vi "S4GUI.vi"(7 "Tab ObsEng":enum32{"Obs", "CCD modes", "Eng"}(tab)) -> ()   [LabVIEW 2018] (continued)
        n2124 = call-dynamic "Read State Machine.vi"("error in (no error)"=w4148, "Device in"=w4150) -> ("error out"=w4159:errorcluster, "State Machine.lvclass"=w4155:refnum<class "State Machine.lvclass">, "Device out"=w4156:refnum<class "Channel.lvclass">)  [unwired: 7 in]
        n2125 = call-dynamic "Read State Machine.vi"("error in (no error)"=w4165, "Device in"=w4167) -> ("error out"=w4176:errorcluster, "State Machine.lvclass"=w4172:refnum<class "State Machine.lvclass">, "Device out"=w4173:refnum<class "Channel.lvclass">)  [unwired: 7 in]
        n2126 = call-dynamic "Read State Machine.vi"("error in (no error)"=w4178, "Device in"=w4180) -> ("error out"=w4191:errorcluster, "State Machine.lvclass"=w4187:refnum<class "State Machine.lvclass">, "Device out"=w4188:refnum<class "Channel.lvclass">)  [unwired: 7 in]
        n2127 = call-dynamic "Write State.vi"("error in (no error)"=w4142, "State"=40, "State Machine in"=w4138) -> ("error out"=w4141:errorcluster, "State Machine out"=w4137:refnum<class "State Machine.lvclass">)  [unwired: 7 in]
        n2128 = call-dynamic "Write State.vi"("error in (no error)"=w4159, "State"=40, "State Machine in"=w4155) -> ("error out"=w4158:errorcluster, "State Machine out"=w4154:refnum<class "State Machine.lvclass">)  [unwired: 7 in]
        n2129 = call-dynamic "Write State.vi"("error in (no error)"=w4176, "State"=40, "State Machine in"=w4172) -> ("error out"=w4175:errorcluster, "State Machine out"=w4171:refnum<class "State Machine.lvclass">)  [unwired: 7 in]
        n2130 = call-dynamic "Write State.vi"("error in (no error)"=w4191, "State"=40, "State Machine in"=w4187) -> ("error out"=w4190:errorcluster, "State Machine out"=w4186:refnum<class "State Machine.lvclass">)  [unwired: 7 in]
        n2131 = call-dynamic "Write State Machine.vi"("error in (no error)"=w4141, "State Machine.lvclass"=w4137, "Device in"=w4139) -> ("error out"=w4135:errorcluster, "Device out"=w4136:refnum<class "Channel.lvclass">)  [unwired: 7 in]
        n2132 = call-dynamic "Write State Machine.vi"("error in (no error)"=w4158, "State Machine.lvclass"=w4154, "Device in"=w4156) -> ("error out"=w4152:errorcluster, "Device out"=w4153:refnum<class "Channel.lvclass">)  [unwired: 7 in]
        n2133 = call-dynamic "Write State Machine.vi"("error in (no error)"=w4175, "State Machine.lvclass"=w4171, "Device in"=w4173) -> ("error out"=w4169:errorcluster, "Device out"=w4170:refnum<class "Channel.lvclass">)  [unwired: 7 in]
        n2134 = call-dynamic "Write State Machine.vi"("error in (no error)"=w4190, "State Machine.lvclass"=w4186, "Device in"=w4188) -> ("error out"=w4184:errorcluster, "Device out"=w4185:refnum<class "Channel.lvclass">)  [unwired: 7 in]
        n2135 = call-dynamic "Write Channel.vi"("error in (no error)"=w4135, "Channel.lvclass"=w4136, "Acquisition in"=w4143) -> ("error out"=w4127:errorcluster, "Acquisition out"=w4128:refnum<class "Acquisition.lvclass">)  [unwired: 7 in]
        n2136 = call-dynamic "Write Channel.vi"("error in (no error)"=w4152, "Channel.lvclass"=w4153, "Acquisition in"=w4160) -> ("error out"=w4145:errorcluster, "Acquisition out"=w4144:refnum<class "Acquisition.lvclass">)  [unwired: 7 in]
        n2137 = call-dynamic "Write Channel.vi"("error in (no error)"=w4169, "Channel.lvclass"=w4170, "Acquisition in"=w4177) -> ("error out"=w4162:errorcluster, "Acquisition out"=w4161:refnum<class "Acquisition.lvclass">)  [unwired: 7 in]
        n2138 = call-dynamic "Write Channel.vi"("error in (no error)"=w4184, "Channel.lvclass"=w4185, "Acquisition in"=w4192) -> ("error out"=w4197:errorcluster, "Acquisition out"=w4198:refnum<class "Acquisition.lvclass">)  [unwired: 7 in]
        n2139 = call-dynamic "Write AcquisitionA.vi"("error in (no error)"=w4197, "Acquisition.lvclass"=w4198, "S4ACS_GUI in"=w4199) -> ("error out"=w4196:errorcluster, "S4ACS_GUI out"=w4202:refnum<class "S4GUI.lvclass">)  [unwired: 7 in]
        n2140 = call "Write AcquisitionB.vi"("error in (no error)"=w4162, "Acquisition.lvclass"=w4161, "S4ACS_GUI in"=w4202) -> ("error out"=w4195:errorcluster, "S4ACS_GUI out"=w4201:refnum<class "S4GUI.lvclass">)  [unwired: 7 in]
        n2141 = call-dynamic "Write AcquisitionC.vi"("error in (no error)"=w4145, "Acquisition.lvclass"=w4144, "S4ACS_GUI in"=w4201) -> ("error out"=w4194:errorcluster, "S4ACS_GUI out"=w4200:refnum<class "S4GUI.lvclass">)  [unwired: 7 in]
        n2142 = call-dynamic "Write AcquisitionD.vi"("error in (no error)"=w4127, "Acquisition.lvclass"=w4128, "S4ACS_GUI in"=w4200) -> ("error out"=w4193:errorcluster, "S4ACS_GUI out"=w4126:refnum<class "S4GUI.lvclass">)  [unwired: 7 in]
        n2143 = Merge Errors(w4196, w4195, w4194, w4193) -> (w4125:errorcluster)
        n2144 = call-dynamic "Write mode EXPOSE.vi"("error in (no error)"=w4125, "mode EXPOSE"=w4120, "S4GUI in"=w4126) -> ("error out"=w4123:errorcluster, "S4GUI out"=w4124:refnum<class "S4GUI.lvclass">)  [unwired: 7 in]
      }
      event "CH1on": Value Change {
        n2145 = event-data() -> ("NewVal"=w4268:bool)  [unwired: 1 in]
        n2146 = call-dynamic "Read AcquisitionA.vi"("error in (no error)"=w4282, "S4ACS_GUI in"=w4283) -> ("error out"=w4274:errorcluster, "Acquisition.lvclass"=w4279:refnum<class "Acquisition.lvclass">, "S4ACS_GUI out"=w4275:refnum<class "S4GUI.lvclass">)  [unwired: 7 in]
        n2147 = call-dynamic "Read Channel.vi"("error in (no error)"=w4274, "Acquisition in"=w4279) -> ("error out"=w4273:errorcluster, "Channel.lvclass"=w4264:refnum<class "Channel.lvclass">, "Acquisition out"=w4278:refnum<class "Acquisition.lvclass">)  [unwired: 7 in]
        n2148 = call-dynamic "Read Stream.vi"("error in (no error)"=w4273, "Server in"=w4278) -> ("error out"=w4266:errorcluster, "Stream.lvclass"=w4267:refnum<class "Stream.lvclass">, "Server out"=w4265:refnum<class "Acquisition.lvclass">)  [unwired: 7 in]
        n2149 = case shown="False" w4268 {
          selector: w4268 -> [w4284 w4306]
          tunnel: [w4290 w4310] -> w4262
          tunnel: w4267 -> [w4299 _]
          tunnel: [w4298 w4313] -> w4261
          tunnel: w4266 -> [w4285 w4307]
          tunnel: w4265 -> [w4286 w4308]
          tunnel: [w4286 w4312] -> w4260
          tunnel: w4264 -> [w4297 w4309]
          tunnel: [w4295 w4309] -> w4259
          tunnel: [w4284 w4306] -> w4263
          frame False {
            # "força FALSE nos parametros do CCD"
            n2150 = call-dynamic "Read Interface.vi"("error in (no error)"=w4285, "Channel in"=w4297) -> ("error out"=w4294:errorcluster, "Interface.lvclass"=w4288:refnum<class "Interface.lvclass">, "Channel out"=w4296:refnum<class "Channel.lvclass">)  [unwired: 7 in]
            n2151 = disable-structure shown="Enabled" {
              disable-tunnel: w4299 -> [w4303 w4305]
              disable-tunnel: [w4302 w4305] -> w4298
              disable-tunnel: [w4301 w4304] -> w4291
              disable-tunnel: w4285 -> [w4300 w4304]
              frame Disabled {
                n2152 = call-dynamic "End.vi"("error in (no error)"=w4300, "Stream in"=w4303) -> ("error out"=w4301:errorcluster, "Stream out"=w4302:refnum<class "Stream.lvclass">)  [unwired: 8 in]
              }
              frame Enabled {
              }
            }
            n2153 = call "Write Checked Params.vi"("error in (no error)"=w4294, "Checked Params"=T14 {"ACQUISITION_MODE"=FALSE, "TRIGGER_MODE"=FALSE, "READ_MODE"=FALSE, "PREAMP"=FALSE, "READOUT_RATE"=FALSE, "VERTICAL_SHIFT_SPEED"=FALSE, "EM_MODE"=FALSE, "EM_GAIN"=FALSE, "SHUTTER_MODE"=FALSE, "SHUTTER_TTL"=FALSE, "SHUTTER_OPENING_TIME"=FALSE, "SHUTTER_CLOSING_TIME"=FALSE, "VBIN"=FALSE, "HBIN"=FALSE, "INITIAL_LINE"=FALSE, "INITIAL_COLUMN"=FALSE, "FINAL_LINE"=FALSE, "FINAL_COLUMN"=FALSE, "FRAME_TRANSFER"=FALSE, "VERTICAL_CLOCK_VOLTAGE"=FALSE, "AD_CHANNEL"=FALSE}, "Interface in"=w4288) -> ("error out"=w4293:errorcluster, "Interface out"=w4287:refnum<class "Interface.lvclass">)  [unwired: 7 in]
            n2154 = call-dynamic "Write Interface.vi"("error in (no error)"=w4293, "Interface.lvclass"=w4287, "Channel in"=w4296) -> ("error out"=w4292:errorcluster, "Channel out"=w4295:refnum<class "Channel.lvclass">)  [unwired: 7 in]
            n2155 = Merge Errors(w4292, w4291) -> (w4290:errorcluster)
          }
          frame True {
            n2156 = call-dynamic "Read Stream.vi"("error in (no error)"=w4307, "Server in"=w4308) -> ("error out"=w4311:errorcluster, "Stream.lvclass"=w4314:refnum<class "Stream.lvclass">, "Server out"=w4312:refnum<class "Acquisition.lvclass">)  [unwired: 7 in]
            n2157 = disable-structure shown="Enabled" {
              disable-tunnel: w4314 -> [w4320 w4330]
              disable-tunnel: [w4319 w4330] -> w4313
              disable-tunnel: w4311 -> [w4317 w4329]
              disable-tunnel: [w4315 w4329] -> w4310
              frame Disabled {
                w4328 = FALSE ("Wait Until Done")
                n2158 = call-dynamic "Read comfile name1.vi"("error in (no error)"=w4317, "Stream in"=w4320) -> ("error out"=w4316:errorcluster, "comfile name1"=w4323:string, "Stream out"=w4318:refnum<class "Stream.lvclass">)  [unwired: 7 in]
                n2159 = call <vilib>:"Application Directory.vi"() -> ("Application Directory"=w4325:path)
                n2160 = Build Path(base path=w4325, name or relative path=w4323) -> (appended path=w4324:path)
                n2161 = Open VI Reference(vi path=w4324, error in (no error)=w4316) -> (vi reference=w4326:refnum<vi>, error out=w4327:errorcluster)  [unwired: 4 in]
                n2162 = invoke class="VI" method="Run VI"(reference=w4326, error in=w4327, "Wait until done"=w4328, "Auto Dispose Ref"=w4328) -> (reference out=w4322:refnum<vi>, error out=w4321:errorcluster)  [unwired: 1 in, 3 out]
                n2163 = call-dynamic "Write commfile ref1.vi"("error in (no error)"=w4321, "commfile ref1"=w4322, "Stream in"=w4318) -> ("error out"=w4315:errorcluster, "Stream out"=w4319:refnum<class "Stream.lvclass">)  [unwired: 7 in]
              }
              frame Enabled {
              }
            }
          }
        }
        n2164 = call-dynamic "Write Stream.vi"("error in (no error)"=w4262, "Stream.lvclass"=w4261, "Server in"=w4260) -> ("error out"=w4272:errorcluster, "Server out"=w4270:refnum<class "Acquisition.lvclass">)  [unwired: 7 in]
        n2165 = call-dynamic "Write enabled.vi"("error in (no error)"=w4272, "enabled"=w4263, "Server in"=w4270) -> ("error out"=w4271:errorcluster, "Server out"=w4269:refnum<class "Acquisition.lvclass">)  [unwired: 7 in]
        n2166 = call-dynamic "Write Channel.vi"("error in (no error)"=w4271, "Channel.lvclass"=w4259, "Acquisition in"=w4269) -> ("error out"=w4277:errorcluster, "Acquisition out"=w4276:refnum<class "Acquisition.lvclass">)  [unwired: 7 in]
        n2167 = call-dynamic "Write AcquisitionA.vi"("error in (no error)"=w4277, "Acquisition.lvclass"=w4276, "S4ACS_GUI in"=w4275) -> ("error out"=w4280:errorcluster, "S4ACS_GUI out"=w4281:refnum<class "S4GUI.lvclass">)  [unwired: 7 in]
      }
      event "CH2on": Value Change {
        n2168 = event-data() -> ("NewVal"=w4332:bool)  [unwired: 1 in]
        n2169 = call "Read AcquisitionB.vi"("error in (no error)"=w4354, "S4ACS_GUI in"=w4355) -> ("error out"=w4346:errorcluster, "Acquisition.lvclass"=w4351:refnum<class "Acquisition.lvclass">, "S4ACS_GUI out"=w4347:refnum<class "S4GUI.lvclass">)  [unwired: 7 in]
        n2170 = call-dynamic "Read Channel.vi"("error in (no error)"=w4346, "Acquisition in"=w4351) -> ("error out"=w4345:errorcluster, "Channel.lvclass"=w4340:refnum<class "Channel.lvclass">, "Acquisition out"=w4350:refnum<class "Acquisition.lvclass">)  [unwired: 7 in]
        n2171 = call-dynamic "Read Stream.vi"("error in (no error)"=w4345, "Server in"=w4350) -> ("error out"=w4336:errorcluster, "Stream.lvclass"=w4333:refnum<class "Stream.lvclass">, "Server out"=w4338:refnum<class "Acquisition.lvclass">)  [unwired: 7 in]
        n2172 = case shown="False" w4332 {
          selector: w4332 -> [w4356 w4378]
          tunnel: [w4362 w4382] -> w4335
          tunnel: w4333 -> [w4371 _]
          tunnel: [w4370 w4385] -> w4334
          tunnel: w4336 -> [w4357 w4379]
          tunnel: w4338 -> [w4358 w4380]
          tunnel: [w4358 w4384] -> w4337
          tunnel: w4340 -> [w4369 w4381]
          tunnel: [w4367 w4381] -> w4339
          tunnel: [w4356 w4378] -> w4331
          frame False {
            # "força FALSE nos parametros do CCD"
            n2173 = call-dynamic "Read Interface.vi"("error in (no error)"=w4357, "Channel in"=w4369) -> ("error out"=w4366:errorcluster, "Interface.lvclass"=w4360:refnum<class "Interface.lvclass">, "Channel out"=w4368:refnum<class "Channel.lvclass">)  [unwired: 7 in]
            n2174 = disable-structure shown="Enabled" {
              disable-tunnel: w4371 -> [w4375 w4377]
              disable-tunnel: [w4374 w4377] -> w4370
              disable-tunnel: [w4373 w4376] -> w4363
              disable-tunnel: w4357 -> [w4372 w4376]
              frame Disabled {
                n2175 = call-dynamic "End.vi"("error in (no error)"=w4372, "Stream in"=w4375) -> ("error out"=w4373:errorcluster, "Stream out"=w4374:refnum<class "Stream.lvclass">)  [unwired: 8 in]
              }
              frame Enabled {
              }
            }
            n2176 = call "Write Checked Params.vi"("error in (no error)"=w4366, "Checked Params"=T14 {"ACQUISITION_MODE"=FALSE, "TRIGGER_MODE"=FALSE, "READ_MODE"=FALSE, "PREAMP"=FALSE, "READOUT_RATE"=FALSE, "VERTICAL_SHIFT_SPEED"=FALSE, "EM_MODE"=FALSE, "EM_GAIN"=FALSE, "SHUTTER_MODE"=FALSE, "SHUTTER_TTL"=FALSE, "SHUTTER_OPENING_TIME"=FALSE, "SHUTTER_CLOSING_TIME"=FALSE, "VBIN"=FALSE, "HBIN"=FALSE, "INITIAL_LINE"=FALSE, "INITIAL_COLUMN"=FALSE, "FINAL_LINE"=FALSE, "FINAL_COLUMN"=FALSE, "FRAME_TRANSFER"=FALSE, "VERTICAL_CLOCK_VOLTAGE"=FALSE, "AD_CHANNEL"=FALSE}, "Interface in"=w4360) -> ("error out"=w4365:errorcluster, "Interface out"=w4359:refnum<class "Interface.lvclass">)  [unwired: 7 in]
            n2177 = call-dynamic "Write Interface.vi"("error in (no error)"=w4365, "Interface.lvclass"=w4359, "Channel in"=w4368) -> ("error out"=w4364:errorcluster, "Channel out"=w4367:refnum<class "Channel.lvclass">)  [unwired: 7 in]
            n2178 = Merge Errors(w4364, w4363) -> (w4362:errorcluster)
          }
          frame True {
            n2179 = call-dynamic "Read Stream.vi"("error in (no error)"=w4379, "Server in"=w4380) -> ("error out"=w4383:errorcluster, "Stream.lvclass"=w4386:refnum<class "Stream.lvclass">, "Server out"=w4384:refnum<class "Acquisition.lvclass">)  [unwired: 7 in]
            n2180 = disable-structure shown="Enabled" {
              disable-tunnel: w4386 -> [w4392 w4402]
              disable-tunnel: [w4391 w4402] -> w4385
              disable-tunnel: w4383 -> [w4389 w4401]
              disable-tunnel: [w4387 w4401] -> w4382
              frame Disabled {
                w4400 = FALSE ("Wait Until Done")
                n2181 = call-dynamic "Read comfile name1.vi"("error in (no error)"=w4389, "Stream in"=w4392) -> ("error out"=w4388:errorcluster, "comfile name1"=w4395:string, "Stream out"=w4390:refnum<class "Stream.lvclass">)  [unwired: 7 in]
                n2182 = call <vilib>:"Application Directory.vi"() -> ("Application Directory"=w4397:path)
                n2183 = Build Path(base path=w4397, name or relative path=w4395) -> (appended path=w4396:path)
                n2184 = Open VI Reference(vi path=w4396, error in (no error)=w4388) -> (vi reference=w4398:refnum<vi>, error out=w4399:errorcluster)  [unwired: 4 in]
                n2185 = invoke class="VI" method="Run VI"(reference=w4398, error in=w4399, "Wait until done"=w4400, "Auto Dispose Ref"=w4400) -> (reference out=w4394:refnum<vi>, error out=w4393:errorcluster)  [unwired: 1 in, 3 out]
                n2186 = call-dynamic "Write commfile ref1.vi"("error in (no error)"=w4393, "commfile ref1"=w4394, "Stream in"=w4390) -> ("error out"=w4387:errorcluster, "Stream out"=w4391:refnum<class "Stream.lvclass">)  [unwired: 7 in]
              }
              frame Enabled {
              }
            }
          }
        }
        n2187 = call-dynamic "Write Stream.vi"("error in (no error)"=w4335, "Stream.lvclass"=w4334, "Server in"=w4337) -> ("error out"=w4342:errorcluster, "Server out"=w4344:refnum<class "Acquisition.lvclass">)  [unwired: 7 in]
        n2188 = call-dynamic "Write enabled.vi"("error in (no error)"=w4342, "enabled"=w4331, "Server in"=w4344) -> ("error out"=w4341:errorcluster, "Server out"=w4343:refnum<class "Acquisition.lvclass">)  [unwired: 7 in]
        n2189 = call-dynamic "Write Channel.vi"("error in (no error)"=w4341, "Channel.lvclass"=w4339, "Acquisition in"=w4343) -> ("error out"=w4349:errorcluster, "Acquisition out"=w4348:refnum<class "Acquisition.lvclass">)  [unwired: 7 in]
        n2190 = call "Write AcquisitionB.vi"("error in (no error)"=w4349, "Acquisition.lvclass"=w4348, "S4ACS_GUI in"=w4347) -> ("error out"=w4352:errorcluster, "S4ACS_GUI out"=w4353:refnum<class "S4GUI.lvclass">)  [unwired: 7 in]
      }
      event "CH3 on": Value Change {
        n2191 = event-data() -> ("NewVal"=w4419:bool)  [unwired: 1 in]
        n2192 = call-dynamic "Read AcquisitionC.vi"("error in (no error)"=w4422, "S4ACS_GUI in"=w4426) -> ("error out"=w4411:errorcluster, "Acquisition.lvclass"=w4416:refnum<class "Acquisition.lvclass">, "S4ACS_GUI out"=w4412:refnum<class "S4GUI.lvclass">)  [unwired: 7 in]
        n2193 = call-dynamic "Read Channel.vi"("error in (no error)"=w4411, "Acquisition in"=w4416) -> ("error out"=w4410:errorcluster, "Channel.lvclass"=w4409:refnum<class "Channel.lvclass">, "Acquisition out"=w4415:refnum<class "Acquisition.lvclass">)  [unwired: 7 in]
        n2194 = call-dynamic "Read Stream.vi"("error in (no error)"=w4410, "Server in"=w4415) -> ("error out"=w4423:errorcluster, "Stream.lvclass"=w4427:refnum<class "Stream.lvclass">, "Server out"=w4421:refnum<class "Acquisition.lvclass">)  [unwired: 7 in]
        n2195 = case shown="False" w4419 {
          selector: w4419 -> [w4428 w4450]
          tunnel: [w4434 w4454] -> w4424
          tunnel: w4427 -> [w4443 _]
          tunnel: [w4442 w4457] -> w4425
          tunnel: w4423 -> [w4429 w4451]
          tunnel: w4421 -> [w4430 w4452]
          tunnel: [w4430 w4456] -> w4420
          tunnel: w4409 -> [w4441 w4453]
          tunnel: [w4439 w4453] -> w4408
          tunnel: [w4428 w4450] -> w4403
          frame False {
            # "força FALSE nos parametros do CCD"
            n2196 = call-dynamic "Read Interface.vi"("error in (no error)"=w4429, "Channel in"=w4441) -> ("error out"=w4438:errorcluster, "Interface.lvclass"=w4432:refnum<class "Interface.lvclass">, "Channel out"=w4440:refnum<class "Channel.lvclass">)  [unwired: 7 in]
            n2197 = disable-structure shown="Disabled" {
              disable-tunnel: w4443 -> [w4447 w4449]
              disable-tunnel: [w4446 w4449] -> w4442
              disable-tunnel: [w4445 w4448] -> w4435
              disable-tunnel: w4429 -> [w4444 w4448]
              frame Disabled {
                n2198 = call-dynamic "End.vi"("error in (no error)"=w4444, "Stream in"=w4447) -> ("error out"=w4445:errorcluster, "Stream out"=w4446:refnum<class "Stream.lvclass">)  [unwired: 8 in]
              }
              frame Enabled {
              }
            }
            n2199 = call "Write Checked Params.vi"("error in (no error)"=w4438, "Checked Params"=T14 {"ACQUISITION_MODE"=FALSE, "TRIGGER_MODE"=FALSE, "READ_MODE"=FALSE, "PREAMP"=FALSE, "READOUT_RATE"=FALSE, "VERTICAL_SHIFT_SPEED"=FALSE, "EM_MODE"=FALSE, "EM_GAIN"=FALSE, "SHUTTER_MODE"=FALSE, "SHUTTER_TTL"=FALSE, "SHUTTER_OPENING_TIME"=FALSE, "SHUTTER_CLOSING_TIME"=FALSE, "VBIN"=FALSE, "HBIN"=FALSE, "INITIAL_LINE"=FALSE, "INITIAL_COLUMN"=FALSE, "FINAL_LINE"=FALSE, "FINAL_COLUMN"=FALSE, "FRAME_TRANSFER"=FALSE, "VERTICAL_CLOCK_VOLTAGE"=FALSE, "AD_CHANNEL"=FALSE}, "Interface in"=w4432) -> ("error out"=w4437:errorcluster, "Interface out"=w4431:refnum<class "Interface.lvclass">)  [unwired: 7 in]
            n2200 = call-dynamic "Write Interface.vi"("error in (no error)"=w4437, "Interface.lvclass"=w4431, "Channel in"=w4440) -> ("error out"=w4436:errorcluster, "Channel out"=w4439:refnum<class "Channel.lvclass">)  [unwired: 7 in]
            n2201 = Merge Errors(w4436, w4435) -> (w4434:errorcluster)
          }
          frame True {
            n2202 = call-dynamic "Read Stream.vi"("error in (no error)"=w4451, "Server in"=w4452) -> ("error out"=w4455:errorcluster, "Stream.lvclass"=w4458:refnum<class "Stream.lvclass">, "Server out"=w4456:refnum<class "Acquisition.lvclass">)  [unwired: 7 in]
            n2203 = disable-structure shown="Enabled" {
              disable-tunnel: w4458 -> [w4464 w4474]
              disable-tunnel: [w4463 w4474] -> w4457
              disable-tunnel: w4455 -> [w4461 w4473]
              disable-tunnel: [w4459 w4473] -> w4454
              frame Disabled {
                w4472 = FALSE ("Wait Until Done")
                n2204 = call-dynamic "Read comfile name1.vi"("error in (no error)"=w4461, "Stream in"=w4464) -> ("error out"=w4460:errorcluster, "comfile name1"=w4467:string, "Stream out"=w4462:refnum<class "Stream.lvclass">)  [unwired: 7 in]
                n2205 = call <vilib>:"Application Directory.vi"() -> ("Application Directory"=w4469:path)
                n2206 = Build Path(base path=w4469, name or relative path=w4467) -> (appended path=w4468:path)
                n2207 = Open VI Reference(vi path=w4468, error in (no error)=w4460) -> (vi reference=w4470:refnum<vi>, error out=w4471:errorcluster)  [unwired: 4 in]
                n2208 = invoke class="VI" method="Run VI"(reference=w4470, error in=w4471, "Wait until done"=w4472, "Auto Dispose Ref"=w4472) -> (reference out=w4466:refnum<vi>, error out=w4465:errorcluster)  [unwired: 1 in, 3 out]
                n2209 = call-dynamic "Write commfile ref1.vi"("error in (no error)"=w4465, "commfile ref1"=w4466, "Stream in"=w4462) -> ("error out"=w4459:errorcluster, "Stream out"=w4463:refnum<class "Stream.lvclass">)  [unwired: 7 in]
              }
              frame Enabled {
              }
            }
          }
        }
        n2210 = call-dynamic "Write Stream.vi"("error in (no error)"=w4424, "Stream.lvclass"=w4425, "Server in"=w4420) -> ("error out"=w4406:errorcluster, "Server out"=w4407:refnum<class "Acquisition.lvclass">)  [unwired: 7 in]
        n2211 = call-dynamic "Write enabled.vi"("error in (no error)"=w4406, "enabled"=w4403, "Server in"=w4407) -> ("error out"=w4404:errorcluster, "Server out"=w4405:refnum<class "Acquisition.lvclass">)  [unwired: 7 in]
        n2212 = call-dynamic "Write Channel.vi"("error in (no error)"=w4404, "Channel.lvclass"=w4408, "Acquisition in"=w4405) -> ("error out"=w4414:errorcluster, "Acquisition out"=w4413:refnum<class "Acquisition.lvclass">)  [unwired: 7 in]
        n2213 = call-dynamic "Write AcquisitionC.vi"("error in (no error)"=w4414, "Acquisition.lvclass"=w4413, "S4ACS_GUI in"=w4412) -> ("error out"=w4417:errorcluster, "S4ACS_GUI out"=w4418:refnum<class "S4GUI.lvclass">)  [unwired: 7 in]
      }
      event "CH4 on": Value Change {
        n2214 = event-data() -> ("NewVal"=w4480:bool)  [unwired: 1 in]
        n2215 = call-dynamic "Read AcquisitionD.vi"("error in (no error)"=w4498, "S4ACS_GUI in"=w4499) -> ("error out"=w4490:errorcluster, "Acquisition.lvclass"=w4495:refnum<class "Acquisition.lvclass">, "S4ACS_GUI out"=w4491:refnum<class "S4GUI.lvclass">)  [unwired: 7 in]
        n2216 = call-dynamic "Read Channel.vi"("error in (no error)"=w4490, "Acquisition in"=w4495) -> ("error out"=w4489:errorcluster, "Channel.lvclass"=w4484:refnum<class "Channel.lvclass">, "Acquisition out"=w4494:refnum<class "Acquisition.lvclass">)  [unwired: 7 in]
        n2217 = call-dynamic "Read Stream.vi"("error in (no error)"=w4489, "Server in"=w4494) -> ("error out"=w4482:errorcluster, "Stream.lvclass"=w4481:refnum<class "Stream.lvclass">, "Server out"=w4483:refnum<class "Acquisition.lvclass">)  [unwired: 7 in]
        n2218 = case shown="False" w4480 {
          selector: w4480 -> [w4500 w4522]
          tunnel: [w4506 w4526] -> w4476
          tunnel: w4481 -> [w4515 _]
          tunnel: [w4514 w4529] -> w4477
          tunnel: w4482 -> [w4501 w4523]
          tunnel: w4483 -> [w4502 w4524]
          tunnel: [w4502 w4528] -> w4478
          tunnel: w4484 -> [w4513 w4525]
          tunnel: [w4511 w4525] -> w4479
          tunnel: [w4500 w4522] -> w4475
          frame False {
            # "força FALSE nos parametros do CCD"
            n2219 = call-dynamic "Read Interface.vi"("error in (no error)"=w4501, "Channel in"=w4513) -> ("error out"=w4510:errorcluster, "Interface.lvclass"=w4504:refnum<class "Interface.lvclass">, "Channel out"=w4512:refnum<class "Channel.lvclass">)  [unwired: 7 in]
            n2220 = disable-structure shown="Disabled" {
              disable-tunnel: w4515 -> [w4519 w4521]
              disable-tunnel: [w4518 w4521] -> w4514
              disable-tunnel: [w4517 w4520] -> w4507
              disable-tunnel: w4501 -> [w4516 w4520]
              frame Disabled {
                n2221 = call-dynamic "End.vi"("error in (no error)"=w4516, "Stream in"=w4519) -> ("error out"=w4517:errorcluster, "Stream out"=w4518:refnum<class "Stream.lvclass">)  [unwired: 8 in]
              }
              frame Enabled {
              }
            }
            n2222 = call "Write Checked Params.vi"("error in (no error)"=w4510, "Checked Params"=T14 {"ACQUISITION_MODE"=FALSE, "TRIGGER_MODE"=FALSE, "READ_MODE"=FALSE, "PREAMP"=FALSE, "READOUT_RATE"=FALSE, "VERTICAL_SHIFT_SPEED"=FALSE, "EM_MODE"=FALSE, "EM_GAIN"=FALSE, "SHUTTER_MODE"=FALSE, "SHUTTER_TTL"=FALSE, "SHUTTER_OPENING_TIME"=FALSE, "SHUTTER_CLOSING_TIME"=FALSE, "VBIN"=FALSE, "HBIN"=FALSE, "INITIAL_LINE"=FALSE, "INITIAL_COLUMN"=FALSE, "FINAL_LINE"=FALSE, "FINAL_COLUMN"=FALSE, "FRAME_TRANSFER"=FALSE, "VERTICAL_CLOCK_VOLTAGE"=FALSE, "AD_CHANNEL"=FALSE}, "Interface in"=w4504) -> ("error out"=w4509:errorcluster, "Interface out"=w4503:refnum<class "Interface.lvclass">)  [unwired: 7 in]
            n2223 = call-dynamic "Write Interface.vi"("error in (no error)"=w4509, "Interface.lvclass"=w4503, "Channel in"=w4512) -> ("error out"=w4508:errorcluster, "Channel out"=w4511:refnum<class "Channel.lvclass">)  [unwired: 7 in]
            n2224 = Merge Errors(w4508, w4507) -> (w4506:errorcluster)
          }
          frame True {
            n2225 = call-dynamic "Read Stream.vi"("error in (no error)"=w4523, "Server in"=w4524) -> ("error out"=w4527:errorcluster, "Stream.lvclass"=w4530:refnum<class "Stream.lvclass">, "Server out"=w4528:refnum<class "Acquisition.lvclass">)  [unwired: 7 in]
            n2226 = disable-structure shown="Enabled" {
              disable-tunnel: w4530 -> [w4536 w4546]
              disable-tunnel: [w4535 w4546] -> w4529
              disable-tunnel: w4527 -> [w4533 w4545]
              disable-tunnel: [w4531 w4545] -> w4526
              frame Disabled {
                w4544 = FALSE ("Wait Until Done")
                n2227 = call-dynamic "Read comfile name1.vi"("error in (no error)"=w4533, "Stream in"=w4536) -> ("error out"=w4532:errorcluster, "comfile name1"=w4539:string, "Stream out"=w4534:refnum<class "Stream.lvclass">)  [unwired: 7 in]
                n2228 = call <vilib>:"Application Directory.vi"() -> ("Application Directory"=w4541:path)
                n2229 = Build Path(base path=w4541, name or relative path=w4539) -> (appended path=w4540:path)
                n2230 = Open VI Reference(vi path=w4540, error in (no error)=w4532) -> (vi reference=w4542:refnum<vi>, error out=w4543:errorcluster)  [unwired: 4 in]
                n2231 = invoke class="VI" method="Run VI"(reference=w4542, error in=w4543, "Wait until done"=w4544, "Auto Dispose Ref"=w4544) -> (reference out=w4538:refnum<vi>, error out=w4537:errorcluster)  [unwired: 1 in, 3 out]
                n2232 = call-dynamic "Write commfile ref1.vi"("error in (no error)"=w4537, "commfile ref1"=w4538, "Stream in"=w4534) -> ("error out"=w4531:errorcluster, "Stream out"=w4535:refnum<class "Stream.lvclass">)  [unwired: 7 in]
              }
              frame Enabled {
              }
            }
          }
        }
        n2233 = call-dynamic "Write Stream.vi"("error in (no error)"=w4476, "Stream.lvclass"=w4477, "Server in"=w4478) -> ("error out"=w4486:errorcluster, "Server out"=w4488:refnum<class "Acquisition.lvclass">)  [unwired: 7 in]
        n2234 = call-dynamic "Write enabled.vi"("error in (no error)"=w4486, "enabled"=w4475, "Server in"=w4488) -> ("error out"=w4485:errorcluster, "Server out"=w4487:refnum<class "Acquisition.lvclass">)  [unwired: 7 in]
        n2235 = call-dynamic "Write Channel.vi"("error in (no error)"=w4485, "Channel.lvclass"=w4479, "Acquisition in"=w4487) -> ("error out"=w4493:errorcluster, "Acquisition out"=w4492:refnum<class "Acquisition.lvclass">)  [unwired: 7 in]
        n2236 = call-dynamic "Write AcquisitionD.vi"("error in (no error)"=w4493, "Acquisition.lvclass"=w4492, "S4ACS_GUI in"=w4491) -> ("error out"=w4496:errorcluster, "S4ACS_GUI out"=w4497:refnum<class "S4GUI.lvclass">)  [unwired: 7 in]
      }
      event "Run WPROT": Value Change {
        n2237 = event-data() -> ("NewVal"=w4554:bool)  [unwired: 1 in]
        n2238 = case shown="True" w4554 {
          tunnel: [u32 0 ("Ciclos  WPROT") "Ciclos  WPROT"] -> w4553
          tunnel: w4550 -> [w4556 w4561]
          tunnel: [w4556 w4560] -> w4549
          tunnel: w4548 -> [w4555 w4559]
          tunnel: [w4555 w4558] -> w4547
          frame False {
          }
          frame True {
            n2239 = call-dynamic "Write Obs_state.vi"("error in (no error)"=w4559, "Obs_state"=u32 350, "S4ACS_GUI in"=w4561) -> ("error out"=w4558:errorcluster, "S4ACS_GUI out"=w4560:refnum<class "S4GUI.lvclass">)  [unwired: 7 in]
          }
        }
        n2240 = call-dynamic "Write cycles wprot.vi"("error in (no error)"=w4547, "cycles wprot"=w4553, "S4GUI in"=w4549) -> ("error out"=w4551:errorcluster, "S4GUI out"=w4552:refnum<class "S4GUI.lvclass">)  [unwired: 7 in]
      }
      event "Start SM": Value Change {
        n2241 = event-data() -> ()  [unwired: 1 in, 6 out]
        n2242 = call-dynamic "Read Obs_state.vi"("error in (no error)"=w4590, "S4ACS_GUI in"=w4591) -> ("error out"=w4577:errorcluster, "Obs_state"=w4588:u32, "S4ACS_GUI out"=w4579:refnum<class "S4GUI.lvclass">)  [unwired: 7 in]
        n2243 = call "Read Instrument.lvclass.vi"("error in (no error)"=w4577, "S4ACS_GUI in"=w4579) -> ("error out"=w4575:errorcluster, "Instrument.lvclass"=w4576:refnum<class "Instrument.lvclass">, "S4ACS_GUI out"=w4578:refnum<class "S4GUI.lvclass">)  [unwired: 7 in]
        n2244 = Not Equal?(x=w4588, y=u32 400) -> (x != y?=w4587:bool)
        n2245 = call-dynamic "Read mode.vi"("error in (no error)"=w4575, "Instrument in"=w4576) -> ("error out"=w4574:errorcluster, "mode"=w4573:bool)  [unwired: 7 in, 1 out]
        n2246 = case shown="True" w4587 {
          tunnel: w4578 -> [w4633 w4721]
          tunnel: w4574 -> [w4634 w4720]
          tunnel: [w4637 w4734] -> w4568
          tunnel: [w4636 w4732] -> w4567
          tunnel: w4584 -> [_ w4741]
          tunnel: w4583 -> [_ w4740]
          tunnel: w4582 -> [_ w4739]
          tunnel: w4581 -> [_ w4738]
          tunnel: w4580 -> [_ w4737]
          tunnel: w4573 -> [_ w4736]
          tunnel: w4572 -> [_ w4711]
          tunnel: w4571 -> [_ w4714]
          tunnel: w4570 -> [_ w4713]
          tunnel: w4569 -> [_ w4712]
          tunnel: ["RESUME SM CLICKED" ("User Event") "START SM" ("User Event")] -> w4564
          frame False {
            # "Obs_state=400 (PAUSED), envia RESUME e vai para Obs_state=500 \npara esperar envio do comando RESUME a todos os canais."
            n2247 = call-dynamic "Write Obs_state.vi"("error in (no error)"=w4634, "Obs_state"=500, "S4ACS_GUI in"=w4633) -> ("error out"=w4638:errorcluster, "S4ACS_GUI out"=w4639:refnum<class "S4GUI.lvclass">)  [unwired: 7 in]
            n2248 = call-dynamic "Read AcquisitionA.vi"("error in (no error)"=w4638, "S4ACS_GUI in"=w4639) -> ("error out"=w4625:errorcluster, "Acquisition.lvclass"=w4629:refnum<class "Acquisition.lvclass">, "S4ACS_GUI out"=w4649:refnum<class "S4GUI.lvclass">)  [unwired: 7 in]
            n2249 = call-dynamic "Read enabled.vi"("error in (no error)"=w4625, "Server in"=w4629) -> ("error out"=w4627:errorcluster, "enabled"=w4626:bool, "Server out"=w4628:refnum<class "Acquisition.lvclass">)  [unwired: 7 in]
            n2250 = call-dynamic "Read Channel.vi"("error in (no error)"=w4627, "Acquisition in"=w4628) -> ("error out"=w4630:errorcluster, "Channel.lvclass"=w4631:refnum<class "Channel.lvclass">, "Acquisition out"=w4648:refnum<class "Acquisition.lvclass">)  [unwired: 7 in]
            n2251 = case shown="True" w4626 {
              tunnel: w4648 -> [w4696 w4709]
              tunnel: [w4696 w4708] -> w4647
              tunnel: [w4695 w4705] -> w4646
              tunnel: w4631 -> [_ w4698]
              tunnel: w4630 -> [w4695 w4697]
              frame False {
              }
              frame True {
                n2252 = call-dynamic "Read State Machine.vi"("error in (no error)"=w4697, "Device in"=w4698) -> ("error out"=w4699:errorcluster, "State Machine.lvclass"=w4700:refnum<class "State Machine.lvclass">, "Device out"=w4704:refnum<class "Channel.lvclass">)  [unwired: 7 in]
                n2253 = call "Next State.vi"("error in (no error)"=w4699, "New_State"=96, "State Machine in"=w4700) -> ("error out"=w4701:errorcluster, "State Machine out"=w4703:refnum<class "State Machine.lvclass">)  [unwired: 7 in]
                n2254 = call-dynamic "Write State Machine.vi"("error in (no error)"=w4701, "State Machine.lvclass"=w4703, "Device in"=w4704) -> ("error out"=w4706:errorcluster, "Device out"=w4707:refnum<class "Channel.lvclass">)  [unwired: 7 in]
                n2255 = call-dynamic "Write Channel.vi"("error in (no error)"=w4706, "Channel.lvclass"=w4707, "Acquisition in"=w4709) -> ("error out"=w4705:errorcluster, "Acquisition out"=w4708:refnum<class "Acquisition.lvclass">)  [unwired: 7 in]
              }
            }
            n2256 = call-dynamic "Write AcquisitionA.vi"("error in (no error)"=w4646, "Acquisition.lvclass"=w4647, "S4ACS_GUI in"=w4649) -> ("error out"=w4645:errorcluster, "S4ACS_GUI out"=w4642:refnum<class "S4GUI.lvclass">)  [unwired: 7 in]
            n2257 = call "Read AcquisitionB.vi"("error in (no error)"=w4645, "S4ACS_GUI in"=w4642) -> ("error out"=w4616:errorcluster, "Acquisition.lvclass"=w4617:refnum<class "Acquisition.lvclass">, "S4ACS_GUI out"=w4618:refnum<class "S4GUI.lvclass">)  [unwired: 7 in]
            n2258 = call-dynamic "Read enabled.vi"("error in (no error)"=w4616, "Server in"=w4617) -> ("error out"=w4620:errorcluster, "enabled"=w4619:bool, "Server out"=w4621:refnum<class "Acquisition.lvclass">)  [unwired: 7 in]
            n2259 = call-dynamic "Read Channel.vi"("error in (no error)"=w4620, "Acquisition in"=w4621) -> ("error out"=w4622:errorcluster, "Channel.lvclass"=w4623:refnum<class "Channel.lvclass">, "Acquisition out"=w4624:refnum<class "Acquisition.lvclass">)  [unwired: 7 in]
            n2260 = case shown="True" w4619 {
              tunnel: w4624 -> [w4681 w4694]
              tunnel: [w4681 w4693] -> w4615
              tunnel: [w4680 w4690] -> w4614
              tunnel: w4623 -> [_ w4683]
              tunnel: w4622 -> [w4680 w4682]
              frame False {
              }
              frame True {
                n2261 = call-dynamic "Read State Machine.vi"("error in (no error)"=w4682, "Device in"=w4683) -> ("error out"=w4684:errorcluster, "State Machine.lvclass"=w4685:refnum<class "State Machine.lvclass">, "Device out"=w4689:refnum<class "Channel.lvclass">)  [unwired: 7 in]
                n2262 = call "Next State.vi"("error in (no error)"=w4684, "New_State"=96, "State Machine in"=w4685) -> ("error out"=w4686:errorcluster, "State Machine out"=w4688:refnum<class "State Machine.lvclass">)  [unwired: 7 in]
                n2263 = call-dynamic "Write State Machine.vi"("error in (no error)"=w4686, "State Machine.lvclass"=w4688, "Device in"=w4689) -> ("error out"=w4691:errorcluster, "Device out"=w4692:refnum<class "Channel.lvclass">)  [unwired: 7 in]
                n2264 = call-dynamic "Write Channel.vi"("error in (no error)"=w4691, "Channel.lvclass"=w4692, "Acquisition in"=w4694) -> ("error out"=w4690:errorcluster, "Acquisition out"=w4693:refnum<class "Acquisition.lvclass">)  [unwired: 7 in]
              }
            }
            n2265 = call "Write AcquisitionB.vi"("error in (no error)"=w4614, "Acquisition.lvclass"=w4615, "S4ACS_GUI in"=w4618) -> ("error out"=w4644:errorcluster, "S4ACS_GUI out"=w4641:refnum<class "S4GUI.lvclass">)  [unwired: 7 in]
            n2266 = call-dynamic "Read AcquisitionC.vi"("error in (no error)"=w4644, "S4ACS_GUI in"=w4641) -> ("error out"=w4604:errorcluster, "Acquisition.lvclass"=w4607:refnum<class "Acquisition.lvclass">, "S4ACS_GUI out"=w4606:refnum<class "S4GUI.lvclass">)  [unwired: 7 in]
            n2267 = call-dynamic "Read enabled.vi"("error in (no error)"=w4604, "Server in"=w4607) -> ("error out"=w4609:errorcluster, "enabled"=w4608:bool, "Server out"=w4610:refnum<class "Acquisition.lvclass">)  [unwired: 7 in]
            n2268 = call-dynamic "Read Channel.vi"("error in (no error)"=w4609, "Acquisition in"=w4610) -> ("error out"=w4611:errorcluster, "Channel.lvclass"=w4612:refnum<class "Channel.lvclass">, "Acquisition out"=w4613:refnum<class "Acquisition.lvclass">)  [unwired: 7 in]
            n2269 = case shown="True" w4608 {
              tunnel: w4613 -> [w4666 w4679]
              tunnel: [w4666 w4678] -> w4605
              tunnel: [w4665 w4675] -> w4603
              tunnel: w4612 -> [_ w4668]
              tunnel: w4611 -> [w4665 w4667]
              frame False {
              }
              frame True {
                n2270 = call-dynamic "Read State Machine.vi"("error in (no error)"=w4667, "Device in"=w4668) -> ("error out"=w4669:errorcluster, "State Machine.lvclass"=w4670:refnum<class "State Machine.lvclass">, "Device out"=w4674:refnum<class "Channel.lvclass">)  [unwired: 7 in]
                n2271 = call "Next State.vi"("error in (no error)"=w4669, "New_State"=96, "State Machine in"=w4670) -> ("error out"=w4671:errorcluster, "State Machine out"=w4673:refnum<class "State Machine.lvclass">)  [unwired: 7 in]
                n2272 = call-dynamic "Write State Machine.vi"("error in (no error)"=w4671, "State Machine.lvclass"=w4673, "Device in"=w4674) -> ("error out"=w4676:errorcluster, "Device out"=w4677:refnum<class "Channel.lvclass">)  [unwired: 7 in]
                n2273 = call-dynamic "Write Channel.vi"("error in (no error)"=w4676, "Channel.lvclass"=w4677, "Acquisition in"=w4679) -> ("error out"=w4675:errorcluster, "Acquisition out"=w4678:refnum<class "Acquisition.lvclass">)  [unwired: 7 in]
              }
            }
            n2274 = call-dynamic "Write AcquisitionC.vi"("error in (no error)"=w4603, "Acquisition.lvclass"=w4605, "S4ACS_GUI in"=w4606) -> ("error out"=w4643:errorcluster, "S4ACS_GUI out"=w4640:refnum<class "S4GUI.lvclass">)  [unwired: 7 in]
            n2275 = call-dynamic "Read AcquisitionD.vi"("error in (no error)"=w4643, "S4ACS_GUI in"=w4640) -> ("error out"=w4594:errorcluster, "Acquisition.lvclass"=w4595:refnum<class "Acquisition.lvclass">, "S4ACS_GUI out"=w4596:refnum<class "S4GUI.lvclass">)  [unwired: 7 in]
            n2276 = call-dynamic "Read enabled.vi"("error in (no error)"=w4594, "Server in"=w4595) -> ("error out"=w4598:errorcluster, "enabled"=w4597:bool, "Server out"=w4599:refnum<class "Acquisition.lvclass">)  [unwired: 7 in]
            n2277 = call-dynamic "Read Channel.vi"("error in (no error)"=w4598, "Acquisition in"=w4599) -> ("error out"=w4600:errorcluster, "Channel.lvclass"=w4601:refnum<class "Channel.lvclass">, "Acquisition out"=w4602:refnum<class "Acquisition.lvclass">)  [unwired: 7 in]
            n2278 = case shown="True" w4597 {
              tunnel: w4602 -> [w4651 w4664]
              tunnel: [w4651 w4663] -> w4593
              tunnel: [w4650 w4660] -> w4592
              tunnel: w4601 -> [_ w4653]
              tunnel: w4600 -> [w4650 w4652]
              frame False {
              }
              frame True {
                n2279 = call-dynamic "Read State Machine.vi"("error in (no error)"=w4652, "Device in"=w4653) -> ("error out"=w4654:errorcluster, "State Machine.lvclass"=w4655:refnum<class "State Machine.lvclass">, "Device out"=w4659:refnum<class "Channel.lvclass">)  [unwired: 7 in]
                n2280 = call "Next State.vi"("error in (no error)"=w4654, "New_State"=96, "State Machine in"=w4655) -> ("error out"=w4656:errorcluster, "State Machine out"=w4658:refnum<class "State Machine.lvclass">)  [unwired: 7 in]
                n2281 = call-dynamic "Write State Machine.vi"("error in (no error)"=w4656, "State Machine.lvclass"=w4658, "Device in"=w4659) -> ("error out"=w4661:errorcluster, "Device out"=w4662:refnum<class "Channel.lvclass">)  [unwired: 7 in]
                n2282 = call-dynamic "Write Channel.vi"("error in (no error)"=w4661, "Channel.lvclass"=w4662, "Acquisition in"=w4664) -> ("error out"=w4660:errorcluster, "Acquisition out"=w4663:refnum<class "Acquisition.lvclass">)  [unwired: 7 in]
              }
            }
            n2283 = call-dynamic "Write AcquisitionD.vi"("error in (no error)"=w4592, "Acquisition.lvclass"=w4593, "S4ACS_GUI in"=w4596) -> ("error out"=w4636:errorcluster, "S4ACS_GUI out"=w4637:refnum<class "S4GUI.lvclass">)  [unwired: 7 in]
          }
          frame True {
            # "vide S4GUI:\nHandleObservationSync.vi"
            # "aba atual em Tab Acq Type"
            n2284 = call "Read Instrument.lvclass.vi"("error in (no error)"=w4720, "S4ACS_GUI in"=w4721) -> ("error out"=w4723:errorcluster, "Instrument.lvclass"=w4725:refnum<class "Instrument.lvclass">, "S4ACS_GUI out"=w4718:refnum<class "S4GUI.lvclass">)  [unwired: 7 in]
            n2285 = call "Read WPROT.vi"("error in (no error)"=w4723, "Instrument in"=w4725) -> ("error out"=w4722:errorcluster, "Opt_Selector.lvclass"=w4724:refnum<class "Opt_Selector.lvclass">)  [unwired: 7 in, 1 out]
            n2286 = call-dynamic "Read sequencia.vi"("error in (no error)"=w4722, "Opt_Selector in"=w4724) -> ("error out"=w4717:errorcluster, "sequencia"=w4719:u16)  [unwired: 7 in, 1 out]
            n2287 = case shown="\"FOCUS\"" w4711 {
              tunnel: [u32 271 ("Obs_state") u32 251 ("Obs_state")] -> w4745
              tunnel: w4718 -> [w4766 w4769]
              tunnel: w4717 -> [w4756 w4768]
              tunnel: [w4764 w4769] -> w4716
              tunnel: [w4755 w4768] -> w4715
              tunnel: w4714 -> [w4763 _]
              tunnel: w4713 -> [w4762 _]
              tunnel: w4712 -> [w4761 _]
              frame "FOCUS" {
                n2288 = call-dynamic "Read TelFocus.lvclass.vi"("error in (no error)"=w4756, "S4GUI in"=w4766) -> ("error out"=w4758:errorcluster, "TelFocus.lvclass"=w4760:refnum<class "TelFocus.lvclass">, "S4GUI out"=w4765:refnum<class "S4GUI.lvclass">)  [unwired: 7 in]
                n2289 = call-dynamic "LoadParam.vi"("#steps"=w4761, "error in (no error)"=w4758, "step"=w4762, "init"=w4763, "TelFocus in"=w4760) -> ("error out"=w4757:errorcluster, "TelFocus out"=w4759:refnum<class "TelFocus.lvclass">)  [unwired: 5 in]
                n2290 = call-dynamic "Write TelFocus.lvclass.vi"("error in (no error)"=w4757, "TelFocus.lvclass"=w4759, "S4GUI in"=w4765) -> ("error out"=w4755:errorcluster, "S4GUI out"=w4764:refnum<class "S4GUI.lvclass">)  [unwired: 7 in]
              }
              frame Default {
              }
            }
            n2291 = case shown="Default" w4711 {
              tunnel: w4736 -> [_ w4751]
              tunnel: [u32 1 ("# Cycles") w4750] -> w4731
              tunnel: [u32 1 w4749] -> w4726
              tunnel: w4719 -> [_ w4748]
              frame "FOCUS" {
                # "Aba FOCUS: Para a sequencia de foco, sempre  #Cycles=1 e #Seqs=1"
              }
              frame Default {
                n2292 = case shown="True" w4751 {
                  tunnel: [0 w4754] -> w4749
                  tunnel: w4748 -> [_ w4753]
                  frame False {
                    # "OV 20230424: \n#SEQ agora armazena as\nposições da lâmina utilizadas.\nNa fotometria, #SEQ=0"
                    # "fotometria:"
                  }
                  frame True {
                    # "OV 20230424: \n#SEQ agora armazena as\nposições da lâmina utilizadas.\nNa polarimetria, #SEQ=WPROT.sequencia"
                    # "polarimetria:"
                    n2293 = To Unsigned Long Integer(number=w4753) -> (unsigned 32bit integer=w4754:u32)
                  }
                }
                n2294 = local read "# Cycles"() -> (w4750:u32)
              }
            }
            n2295 = call-dynamic "Write Obs_state.vi"("error in (no error)"=w4715, "Obs_state"=w4745, "S4ACS_GUI in"=w4716) -> ("error out"=w4744:errorcluster, "S4ACS_GUI out"=w4743:refnum<class "S4GUI.lvclass">)  [unwired: 7 in]
            n2296 = stacked-sequence {
              seq-local: [w4799 _ _ _] -> [_ w4885 _ _]
              seq-local: [w4798 _ _ _] -> [_ w4884 _ _]
              seq-local: [_ w4883 _ _] -> [_ _ w4946 _]
              seq-local: [_ w4882 _ _] -> [_ _ w4945 _]
              seq-local: [_ _ w4944 _] -> [_ _ _ w5007]
              seq-local: [_ _ w4943 _] -> [_ _ _ w5006]
              tunnel: w4744 -> [w4817 _ _ _]
              tunnel: w4743 -> [w4816 _ _ _]
              tunnel: [_ _ _ w5005] -> w4728
              tunnel: [_ _ _ w5004] -> w4730
              tunnel: w4741 -> [w4797 w4881 w4942 w5003]
              tunnel: w4740 -> [w4796 w4880 w4918 w4979]
              tunnel: w4739 -> [w4795 w4856 w4917 w4978]
              tunnel: w4738 -> [w4794 w4855 w4916 w4977]
              tunnel: w4737 -> [w4789 w4850 w4911 w4972]
              tunnel: w4731 -> [w4786 w4847 w4908 w4969]
              tunnel: w4726 -> [w4781 w4842 w4903 w4964]
              tunnel: w4711 -> [w4775 w4838 w4899 w4958]
              frame #0 {
                # "object"
                # "suffix"
                # "obsType"
                n2297 = local read "Exptime ch1"() -> (w4776:dbl)
                n2298 = call-dynamic "Read AcquisitionA.vi"("error in (no error)"=w4817, "S4ACS_GUI in"=w4816) -> ("error out"=w4815:errorcluster, "Acquisition.lvclass"=w4814:refnum<class "Acquisition.lvclass">, "S4ACS_GUI out"=w4804:refnum<class "S4GUI.lvclass">)  [unwired: 7 in]
                n2299 = call-dynamic "Read Channel.vi"("error in (no error)"=w4815, "Acquisition in"=w4814) -> ("error out"=w4812:errorcluster, "Channel.lvclass"=w4813:refnum<class "Channel.lvclass">, "Acquisition out"=w4803:refnum<class "Acquisition.lvclass">)  [unwired: 7 in]
                n2300 = local read "Exp ch1"() -> (w4801:u32)
                n2301 = call-dynamic "Read Interface.vi"("error in (no error)"=w4812, "Channel in"=w4813) -> ("error out"=w4824:errorcluster, "Interface.lvclass"=w4810:refnum<class "Interface.lvclass">, "Channel out"=w4811:refnum<class "Channel.lvclass">)  [unwired: 7 in]
                n2302 = call "Write Exposure Time.vi"("error in (no error)"=w4824, "Exposure Time"=w4776, "Interface in"=w4810) -> ("error out"=w4777:errorcluster, "Interface out"=w4780:refnum<class "Interface.lvclass">)  [unwired: 7 in]
                n2303 = case shown="Default" w4775 {
                  tunnel: w4780 -> [w4826 w4831]
                  tunnel: [w4826 w4830] -> w4779
                  tunnel: [w4825 w4829] -> w4778
                  tunnel: w4777 -> [w4825 w4828]
                  tunnel: w4776 -> [_ w4827]
                  frame "ZERO" {
                  }
                  frame Default {
                    n2304 = call-dynamic "Write prev ExpTime.vi"("error in (no error)"=w4828, "prev ExpTime"=w4827, "Interface in"=w4831) -> ("error out"=w4829:errorcluster, "Interface out"=w4830:refnum<class "Interface.lvclass">)  [unwired: 7 in]
                  }
                }
                n2305 = call-dynamic "Write Suffix.vi"("error in (no error)"=w4778, "Suffix"=w4797, "Interface in"=w4779) -> ("error out"=w4823:errorcluster, "Interface out"=w4809:refnum<class "Interface.lvclass">)  [unwired: 7 in]
                n2306 = call-dynamic "Write ObsType.vi"("error in (no error)"=w4823, "ObsType"=w4795, "Interface in"=w4809) -> ("error out"=w4822:errorcluster, "Interface out"=w4808:refnum<class "Interface.lvclass">)  [unwired: 7 in]
                n2307 = call-dynamic "Write Object.vi"("error in (no error)"=w4822, "Object"=w4794, "Interface in"=w4808) -> ("error out"=w4821:errorcluster, "Interface out"=w4807:refnum<class "Interface.lvclass">)  [unwired: 7 in]
                n2308 = call-dynamic "Write Comments.vi"("error in (no error)"=w4821, "Comments"=w4796, "Interface in"=w4807) -> ("error out"=w4820:errorcluster, "Interface out"=w4806:refnum<class "Interface.lvclass">)  [unwired: 7 in]
                n2309 = call-dynamic "Write DS9.vi"("error in (no error)"=w4820, "DS9"="F", "Interface in"=w4806) -> ("error out"=w4791:errorcluster, "Interface out"=w4793:refnum<class "Interface.lvclass">)  [unwired: 7 in]
                n2310 = call-dynamic "Write Observer.vi"("error in (no error)"=w4791, "Observer"=w4789, "Interface in"=w4793) -> ("error out"=w4790:errorcluster, "Interface out"=w4792:refnum<class "Interface.lvclass">)  [unwired: 7 in]
                n2311 = call-dynamic "Write # Images.vi"("error in (no error)"=w4790, "# Images"=w4801, "Interface in"=w4792) -> ("error out"=w4818:errorcluster, "Interface out"=w4805:refnum<class "Interface.lvclass">)  [unwired: 7 in]
                n2312 = property on="Exposures Done ch1" class="Slide (strict)"("Scale.Maximum"=w4801, "Scale.Minimum"=0.0 ("Scale.Range:Minimum")) -> ()  [unwired: 2 in, 2 out]
                n2313 = property on="Exposure Time ch1" class="Slide (strict)"("Scale.Maximum"=w4776, "Scale.Minimum"=0.0 ("Scale.Range:Minimum")) -> ()  [unwired: 2 in, 2 out]
                n2314 = call-dynamic "Write Interface.vi"("error in (no error)"=w4818, "Interface.lvclass"=w4805, "Channel in"=w4811) -> ("error out"=w4788:errorcluster, "Channel out"=w4787:refnum<class "Channel.lvclass">)  [unwired: 7 in]
                n2315 = call-dynamic "Write ciclos.vi"("error in (no error)"=w4788, "ciclos"=w4786, "Channel in"=w4787) -> ("error out"=w4783:errorcluster, "Channel out"=w4785:refnum<class "Channel.lvclass">)  [unwired: 7 in]
                n2316 = call-dynamic "Write sequencias.vi"("error in (no error)"=w4783, "sequencias"=w4781, "Channel in"=w4785) -> ("error out"=w4782:errorcluster, "Channel out"=w4784:refnum<class "Channel.lvclass">)  [unwired: 7 in]
                n2317 = call-dynamic "Write Channel.vi"("error in (no error)"=w4782, "Channel.lvclass"=w4784, "Acquisition in"=w4803) -> ("error out"=w4772:errorcluster, "Acquisition out"=w4774:refnum<class "Acquisition.lvclass">)  [unwired: 7 in]
                n2318 = call-dynamic "CalcCubeDuration.vi"("error in (no error)"=w4772, "Acquisition in"=w4774) -> ("error out"=w4771:errorcluster, "Acquisition out"=w4773:refnum<class "Acquisition.lvclass">)  [unwired: 8 in]
                n2319 = call-dynamic "Write AcquisitionA.vi"("error in (no error)"=w4771, "Acquisition.lvclass"=w4773, "S4ACS_GUI in"=w4804) -> ("error out"=w4798:errorcluster, "S4ACS_GUI out"=w4799:refnum<class "S4GUI.lvclass">)  [unwired: 7 in]
              }
              frame #1 {
                # "object"
                # "suffix"
                # "obsType"
                n2320 = call "Read AcquisitionB.vi"("error in (no error)"=w4884, "S4ACS_GUI in"=w4885) -> ("error out"=w4867:errorcluster, "Acquisition.lvclass"=w4868:refnum<class "Acquisition.lvclass">, "S4ACS_GUI out"=w4878:refnum<class "S4GUI.lvclass">)  [unwired: 7 in]
                n2321 = local read "Exptime ch2"() -> (w4839:dbl)
                n2322 = call-dynamic "Read Channel.vi"("error in (no error)"=w4867, "Acquisition in"=w4868) -> ("error out"=w4870:errorcluster, "Channel.lvclass"=w4869:refnum<class "Channel.lvclass">, "Acquisition out"=w4879:refnum<class "Acquisition.lvclass">)  [unwired: 7 in]
                n2323 = call-dynamic "Read Interface.vi"("error in (no error)"=w4870, "Channel in"=w4869) -> ("error out"=w4861:errorcluster, "Interface.lvclass"=w4872:refnum<class "Interface.lvclass">, "Channel out"=w4871:refnum<class "Channel.lvclass">)  [unwired: 7 in]
